vi "Logging Filter by Path.vi"(1 "Path":string, 2 "In":T1) -> (0 "Out":T1)   [LabVIEW 2012, in "femtoRoboLib.lvlib"]
uses:
  femtoRoboLib.lvlib
  Controls/Log Entry - Full Block.ctl
  Controls/Log Entry.ctl
  Controls/Log Value Type.ctl
  Controls/Log Value Cluster.ctl
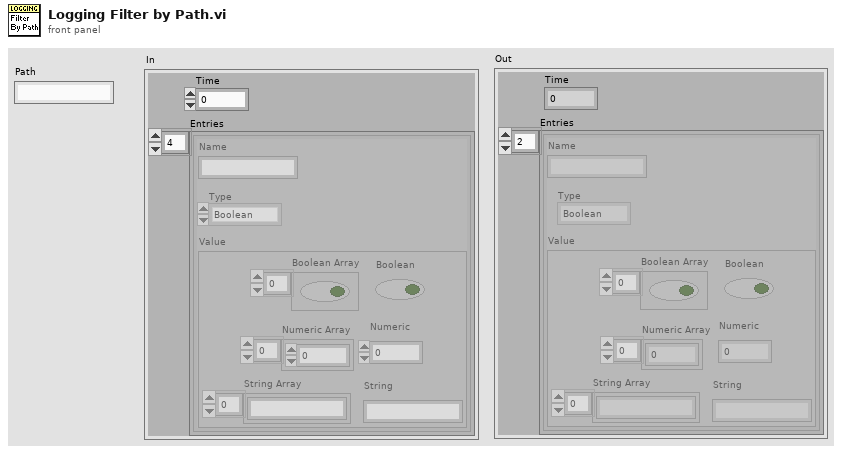
[diagram p1: front panel]
types:
  T1 = typedef "femtoRoboLib.lvlib/Log Entry - Full Block.ctl" = cluster{"Entries":T2[], "Time":u32}
  T2 = typedef "femtoRoboLib.lvlib/Log Entry.ctl" = cluster{"Name":string, "Type":T3, "Value":T4}
  T3 = typedef "femtoRoboLib.lvlib/Log Value Type.ctl" = enum16{"Boolean", "Numeric", "String", "Boolean Array", "Numeric Array", "String Array"}
  T4 = typedef "femtoRoboLib.lvlib/Log Value Cluster.ctl" = cluster{"Boolean Array":bool[], "Boolean":bool, "Numeric Array":dbl[], "Numeric":dbl, "String Array":string[], "String":string}
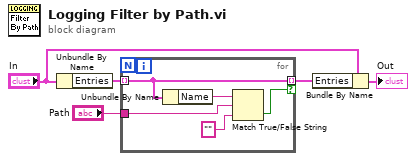
[diagram p0: block diagram]
diagram:
  n1 = Unbundle By Name("In") -> ("Entries"=w5:T2[])
  n2 = for {
    tunnel: w5 -> [w10] mode=indexing
    tunnel: [w10] -> w3 mode=indexing if=w7
    tunnel: "Path" -> [w8]
    n3 = Unbundle By Name(w10) -> ("Name"=w9:string)
    n4 = Match True/False String(2:"" ("false string"), 3:w8, 4:w9) -> (0:w7:bool)  [unwired: 1 out]
  }
  n5 = Bundle By Name(cluster="In", "Entries"=w3) -> (→"Out":T1)
